vi "ArrayRead_D.140620.vi"(0 "Current (or Cued Trial Parameters)":dbl[](array[numeric])) -> (4 "Value 0":dbl, 6 "Value 1":dbl, 8 "Value 2":dbl, 10 "Value 3":dbl, 11 "Value 8":dbl, 12 "Value 7":dbl, 13 "Value 6":dbl, 14 "Value 5":dbl, 15 "Value 4":dbl)   [LabVIEW 2013]
doc: "This VI allows you to access the first 9 elements in a double array. If there are less elements, you will get the default value of zero in return."
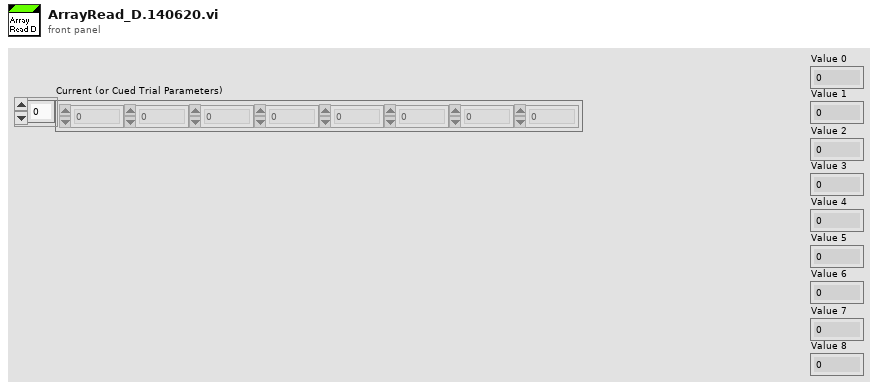
[diagram p1: front panel]
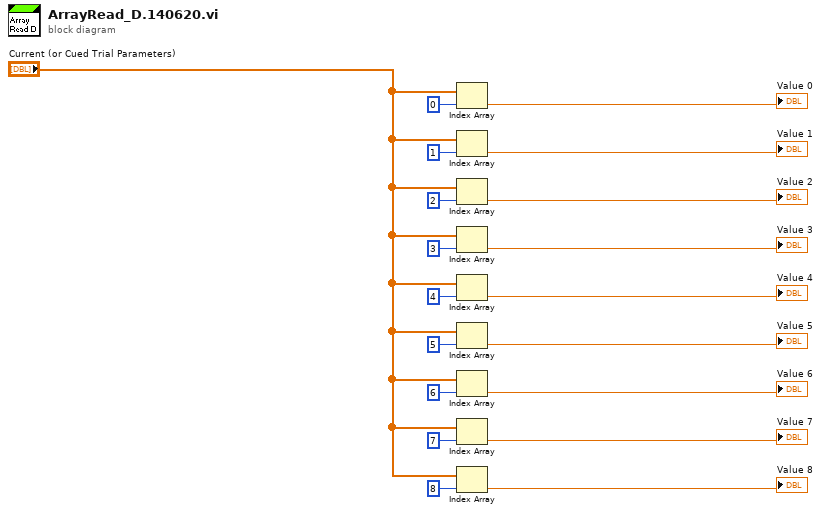
[diagram p0: block diagram]
diagram:
  n1 = Index Array(array="Current (or Cued Trial Parameters)", index=0) -> (element=→"Value 0":dbl)
  n2 = Index Array(array="Current (or Cued Trial Parameters)", index=1) -> (element=→"Value 1":dbl)
  n3 = Index Array(array="Current (or Cued Trial Parameters)", index=2) -> (element=→"Value 2":dbl)
  n4 = Index Array(array="Current (or Cued Trial Parameters)", index=3) -> (element=→"Value 3":dbl)
  n5 = Index Array(array="Current (or Cued Trial Parameters)", index=4) -> (element=→"Value 4":dbl)
  n6 = Index Array(array="Current (or Cued Trial Parameters)", index=5) -> (element=→"Value 5":dbl)
  n7 = Index Array(array="Current (or Cued Trial Parameters)", index=6) -> (element=→"Value 6":dbl)
  n8 = Index Array(array="Current (or Cued Trial Parameters)", index=7) -> (element=→"Value 7":dbl)
  n9 = Index Array(array="Current (or Cued Trial Parameters)", index=8) -> (element=→"Value 8":dbl)
